vi "StageJog.vi"(8 "error in (no error)":errorcluster, 9 "direction":i32(ring)=1 items=["Forward"=1, "Backward"=2], 10 "Stage Select":T1, 11 "Device In":T2) -> (0 "error out":errorcluster)   [LabVIEW 2014]
doc: "Jog the stage with a used defined step size"
uses:
  TypeDef/StageDeviceOut.ctl
  C:/Users/light/Desktop/Peng/Raman/dll/ThorLabs.MotionControl.KCube.DCServoCLI.dll
  dll/ThorLabs.MotionControl.KCube.DCServoCLI.dll
  TypeDef/StageSelect.ctl
panel:
  # "Jog the stage with a used defined step size"
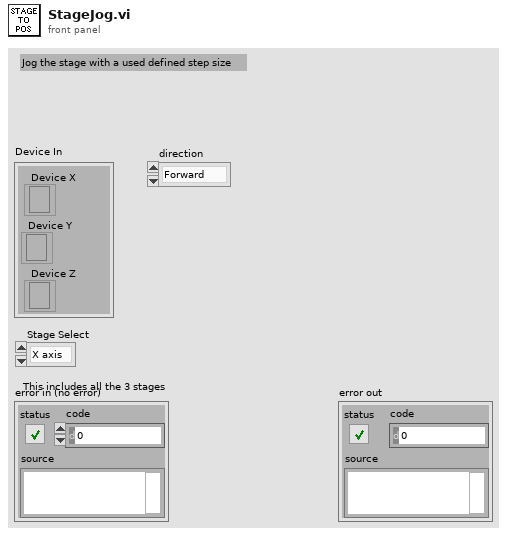
[diagram p1: front panel]
types:
  T1 = typedef "StageSelect.ctl" = enum16{"X axis", "Y axis", "Z axis"}
  T2 = typedef "StageDeviceOut.ctl" = cluster{"Device Z":refnum<k24>, "Device X":refnum<k24>, "Device Y":refnum<k24>}
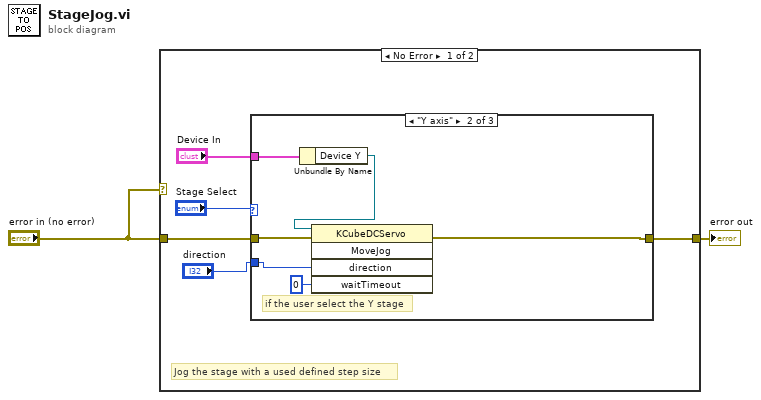
[diagram p0: block diagram]
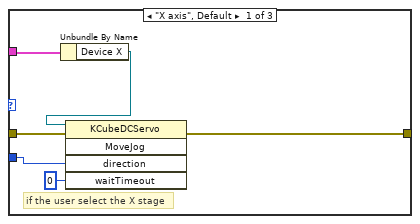
[diagram p2: hidden frame]
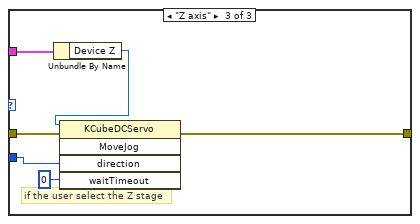
[diagram p3: hidden frame]
diagram:
  n1 = case shown="No Error" "error in (no error)" {
    tunnel: "error in (no error)" -> [w7 w26]
    tunnel: [w5 w26] -> w1
    frame No Error {
      # "Jog the stage with a used defined step size"
      n2 = case shown="\"Y axis\"" "Stage Select" {
        tunnel: w7 -> [w11 w17 w23]
        tunnel: [w10 w15 w22] -> w5
        tunnel: "Device In" -> [w13 w19 w24]
        tunnel: "direction" -> [w9 w16 w21]
        frame "X axis", Default {
          # "if the user select the X stage"
          n3 = Unbundle By Name(w13) -> ("Device X"=w12:refnum<k24>)
          n4 = invoke class="KCubeDCServo" method="MoveJog"(reference=w12, error in=w11, "direction"=w9, "waitTimeout"=0) -> (error out=w10:errorcluster)  [unwired: 1 in, 4 out]
        }
        frame "Y axis" {
          # "if the user select the Y stage"
          n5 = Unbundle By Name(w19) -> ("Device Y"=w18:refnum<k24>)
          n6 = invoke class="KCubeDCServo" method="MoveJog"(reference=w18, error in=w17, "direction"=w16, "waitTimeout"=0) -> (error out=w15:errorcluster)  [unwired: 1 in, 4 out]
        }
        frame "Z axis" {
          # "if the user select the Z stage"
          n7 = Unbundle By Name(w24) -> ("Device Z"=w25:refnum<k24>)
          n8 = invoke class="KCubeDCServo" method="MoveJog"(reference=w25, error in=w23, "direction"=w21, "waitTimeout"=0) -> (error out=w22:errorcluster)  [unwired: 1 in, 4 out]
        }
      }
    }
    frame Error {
    }
  }
  "error out" <- w1
